vi "init.vi"(5 "Scan control":refnum<vi>, 6 "Setup control":refnum<vi>, 7 "Session control":refnum<vi>, 8 "error in (no error)":errorcluster, 10 "Session - Pipeline":path=path "Z:/users/Manolis/Labview/Cajal/Cajal-manolis.dsn", 11 "Experiment in":refnum<class "Experiment.lvclass">) -> (0 "error out":errorcluster, 3 "Experiment out":refnum<class "Experiment.lvclass">)   [LabVIEW 2014, in "Experiment.lvclass"]
uses:
  Experiment.lvclass
  Experiment.lvclass/Experiment.ctl
  Database/Database.lvclass
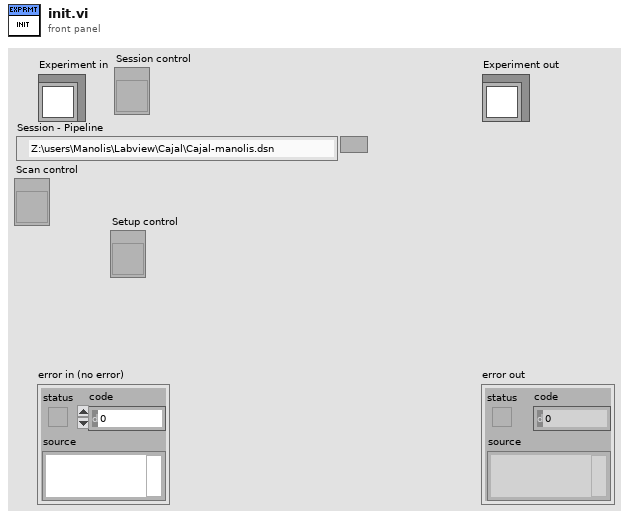
[diagram p1: front panel]
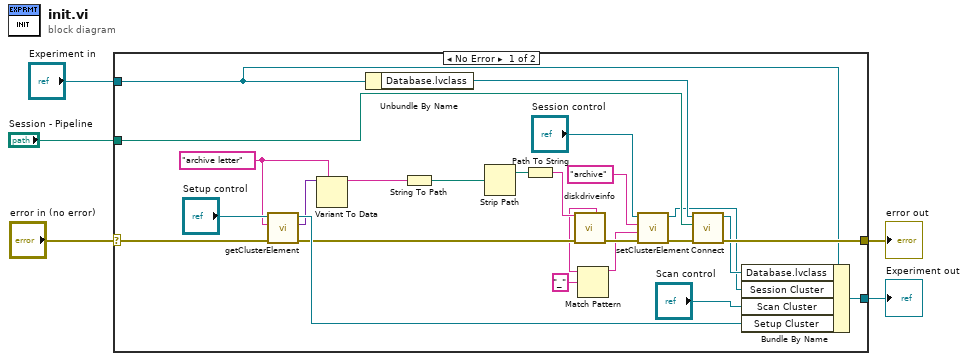
[diagram p0: block diagram]
diagram:
  n1 = case shown="No Error" "error in (no error)" {
    selector: "error in (no error)" -> [w19 w32]
    tunnel: [w29 w32] -> w4
    tunnel: [w25 w31] -> w2
    tunnel: "Experiment in" -> [w27 w31]
    tunnel: "Session - Pipeline" -> [w28 _]
    frame No Error {
      w13 = "archive letter" ("Label.Text")
      n2 = call "getClusterElement.vi"("error in (no error)"=w19, "Label.Text"=w13, "reference"="Setup control") -> ("error out"=w17:errorcluster, "Value"=w14:variant, "reference 2"=w21:refnum<vi>)  [unwired: 6 in]
      n3 = Variant To Data(type=w13, Variant=w14) -> (data=w12:string)  [unwired: 1 in, 1 out]
      n4 = Unbundle By Name(w27) -> ("Database.lvclass"=w30:refnum<class "Database.lvclass">)
      n5 = String To Path(string=w12) -> (path=w11:path)
      n6 = Strip Path(path=w11) -> (stripped path=w10:path)  [unwired: 1 out]
      n7 = Path To String(path=w10) -> (string=w9:string)
      n8 = call "diskdriveinfo.vi"("Drive Letter"=w9, "error in (no error)"=w17) -> ("drive name"=w8:string, "error out"=w16:errorcluster)  [unwired: 4 in, 8 out]
      n9 = Match Pattern(string=w8, regular expression="_") -> (before substring=w6:string)  [unwired: 1 in, 3 out]
      n10 = call "setClusterElement.vi"("error in (no error)"=w16, "Value"=w6, "Label.Text"="archive", "reference"="Session control") -> ("error out"=w18:errorcluster, "reference 2"=w20:refnum<vi>)  [unwired: 6 in]
      n11 = call-dynamic "Connect.vi"("error in (no error)"=w18, "Session - Pipeline"=w28, "Database in"=w30) -> ("error out"=w29:errorcluster, "Database out"=w26:refnum<class "Database.lvclass">)  [unwired: 7 in]
      n12 = Bundle By Name(cluster=w27, "Database.lvclass"=w26, "Session Cluster"=w20, "Scan Cluster"="Scan control", "Setup Cluster"=w21) -> (w25:refnum<class "Experiment.lvclass">)
    }
    frame Error {
    }
  }
  "error out" <- w4
  "Experiment out" <- w2
